vi "Find.vi"(2 "Key":string, 3 "Data":T1(array[cluster])) -> (0 "Found?":bool, 1 "Value":refnum<class "Abstract.lvclass">)   [LabVIEW 2018, in "Toolkit.lvlib" / "Loaders.lvlib" / "Data.lvclass"]
uses:
  Data.lvclass
  Data/Abstract/Abstract.lvclass
  Data/Null/Null.lvclass
  D:/Users/cfield/Code/Field R&D Services/Mustache/trunk/src/Toolkit/Data/Abstract/Abstract.lvclass
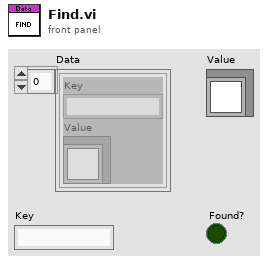
[diagram p1: front panel]
types:
  T1 = cluster{"Key":string, "Value":refnum<class "Abstract.lvclass">}[]
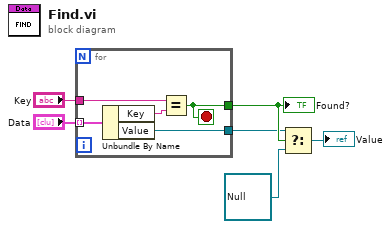
[diagram p0: block diagram]
diagram:
  n1 = for {
    tunnel: "Data" -> [w11] mode=indexing
    tunnel: "Key" -> [w10]
    tunnel: [w8] -> w2
    tunnel: [w7] -> w4
    stop <- w7 stop-if-true
    n2 = Unbundle By Name(w11) -> ("Key"=w9:string, "Value"=w8:refnum<class "Abstract.lvclass">)
    n3 = Equal?(x=w10, y=w9) -> (x = y?=w7:bool)
  }
  "Found?" <- w4
  n4 = Select(t=w2, s=w4, f=refnum<class "Null.lvclass"> refnum ("Toolkit.lvlib:Data.lvlib:Null.lvclass")) -> (s? t:f=→"Value":refnum<class "Abstract.lvclass">)
